vi "Simple UDP - Receiver.vi"() -> ()   [LabVIEW 2023]
doc: "The UDP protocol differs from TCP in that there is no error-checking with the packets of information that are sent, and thus no guarantee whatsoever that an intended recipient will actually receive a given piece of data.\n\nUDP does offer the ability to \"broadcast\" data across a network--simply specify an IP Address of all ones (255.255.255.255) to attempt to broadcast information network-wide. Keep in mind that routers and other network hardware will generally refuse to forward the broadcast beyond certain points, so the extent of the broadcast will in practice be limited."
panel:
  out "Camera":u8
  in  "Stop":bool
  # "Overview: Demonstrates the use of the UDP functions to receive data over a UDP connection.\nInstructions:\n1. Ensure Simple UDP - Sender.vi is already running.\n2. Run the VI.\n3. Click Stop to stop the VI."
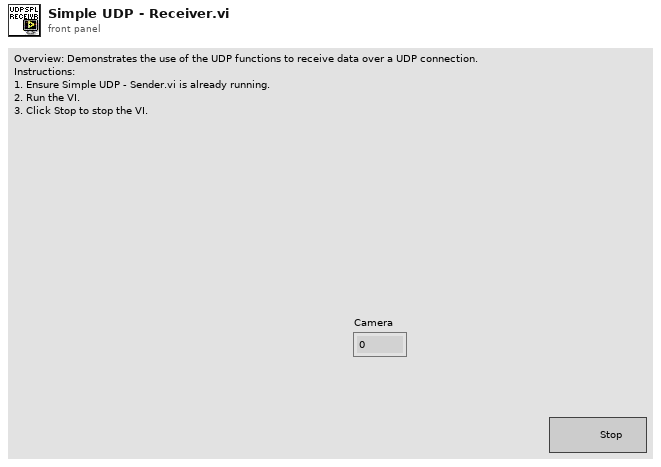
[diagram p1: front panel]
types:
  T1 = typedef "Event Setup Types.ctl" = enum16{"Default", "Camera Loop Started", "Close Settings", "GreyScale", "Open Front Panel", "Save Data", "Exit"}
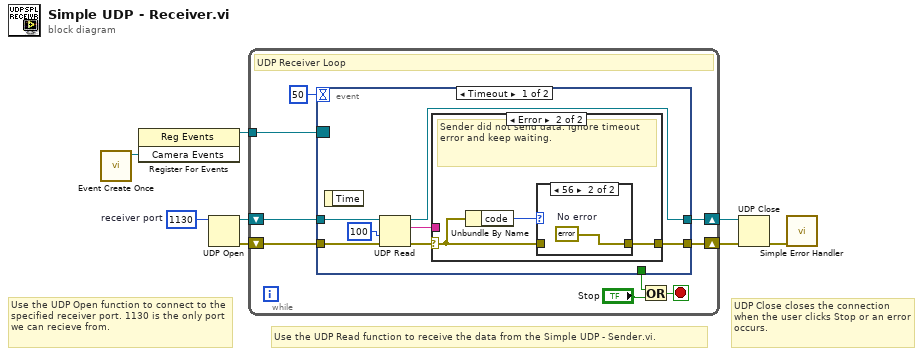
[diagram p0: block diagram]
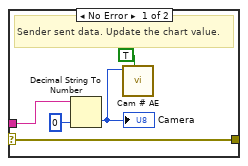
[diagram p2: hidden frame]
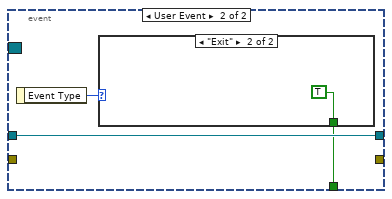
[diagram p4: hidden frame]
diagram:
  w3 = u16 1130  # receiver port
  # "UDP Close closes the connection when the user clicks Stop or an error occurs."
  # "Use the UDP Open function to connect to the specified receiver port. 1130 is the only port we can recieve from."
  # "Use the UDP Read function to receive the data from the Simple UDP - Sender.vi."
  n1 = call "Event Create Once.vi"() -> ("Camera Events"=w2:refnum<user-event>)  [unwired: 10 in, 1 out]
  n2 = register-events(w2) -> (reference out=w1:refnum<event-registration>)  [unwired: 2 in, 1 out]
  n3 = UDP Open(11:w3) -> (port=w4:refnum<k16>, 0:w5:errorcluster)  [unwired: 4 in, 1 out]
  n4 = while {
    shift-right: [w15] -> w8
    shift-left: w4 -> [w17]
    shift-right: [w12] -> w6
    shift-left: w5 -> [w16]
    tunnel: w1 -> [w13]
    stop <- w10 stop-if-true
    # "UDP Receiver Loop"
    n5 = event shown="[0] Timeout" {
      selector: w13 -> [_ _]
      dyn-events: _ -> [_ _]
      timeout: 50 -> [_ _]
      tunnel: w17 -> [w24 w37]
      tunnel: w16 -> [w23 _]
      tunnel: [w19 w37] -> w15
      tunnel: [w18 _] -> w12
      tunnel: [_ w35] -> w9
      event Timeout {
        n6 = event-data() -> ()  [unwired: 1 in, 1 out]
        n7 = UDP Read(connection ID=w24, timeout ms (25000)=100, 8:w23) -> (data out=w21:string, error out=w20:errorcluster, 3:w19:refnum<k16>)  [unwired: 3 out]
        n8 = case shown="Error" w20 {
          selector: w20 -> [w28 w31]
          tunnel: w21 -> [w29 _]
          tunnel: [w28 w30] -> w18
          frame No Error {
            # "Sender sent data. Update the chart value."
            n9 = Decimal String To Number(string=w29, default (0L)=u8 0 ("default (0 I32)")) -> (number=w25:u8)  [unwired: 1 in, 1 out]
            "Camera" <- w25
            n10 = call "Cam # AE.vi"("Update?"=TRUE, "Ball # In"=w25) -> ()  [unwired: 9 in, 1 out]
          }
          frame Error {
            # "Sender did not send data. Ignore timeout error and keep waiting."
            n11 = Unbundle By Name(w31) -> ("code"=w32:i32)
            n12 = case shown="56" w32 {
              tunnel: w31 -> [w33 _]
              tunnel: [w33 w34] -> w30
              frame Default {
              }
              frame 56 {
                w34 = errorcluster {"status"=FALSE, "code"=0, "source"=""}  # No error
              }
            }
          }
        }
      }
      event User Event {
        n13 = event-data() -> ("Event Type"=w36:T1)  [unwired: 1 in]
        n14 = case shown="\"Exit\"" w36 {
          tunnel: [_ TRUE] -> w35
          frame "Default", Default {
          }
          frame "Exit" {
          }
        }
      }
    }
    n15 = Or(x=w9, y="Stop") -> (x .or. y?=w10:bool)
  }
  n16 = UDP Close(connection ID=w8, 8:w6) -> (error out=w7:errorcluster)  [unwired: 1 out]
  n17 = call <vilib>:"Simple Error Handler.vi"("error in (no error)"=w7) -> ()  [unwired: 1 in, 8 out]
